vi "ztscopeM Download Record.vi"(0 "Instrument Handle In":i32, 1 "startTime":dbl format="%^#_6g", 5 "Source":i32(ring) items=["Input Channel 1", "Input Channel 2", "Input Channel 3", "Input Channel 4", "Calc Channel 1", "Calc Channel 2", "Calc Channel 3", "Calc Channel 4", "Ref Channel 1", "Ref Channel 2", "Ref Channel 3", "Ref Channel 4"], 7 "Points":i32=1000, 9 "Transfer Type":i32(ring)=2 items=["s8", "s16", "s32", "f32", "f64"], 11 "error in":errorcluster, 12 "stopTime":dbl format="%^#_6g") -> (3 "F64 Wave":dbl[](array[numeric]), 4 "Instrument Handle Out":i32, 6 "S8 Wave":i8[](array[numeric]), 8 "S16 Wave":i16[](array[numeric]), 10 "S32 Wave":i32[](array[numeric]), 14 "F32 Wave":sgl[](array[numeric]), 15 "error out":errorcluster)   [LabVIEW 2013]
doc: "Read the waveform in the source channel. The returned data format depends on the Transfer Type. Use \"Read Waveform Preamble\" to get the appropriate time and magnitude bases."
uses:
  ztscopeM.dll
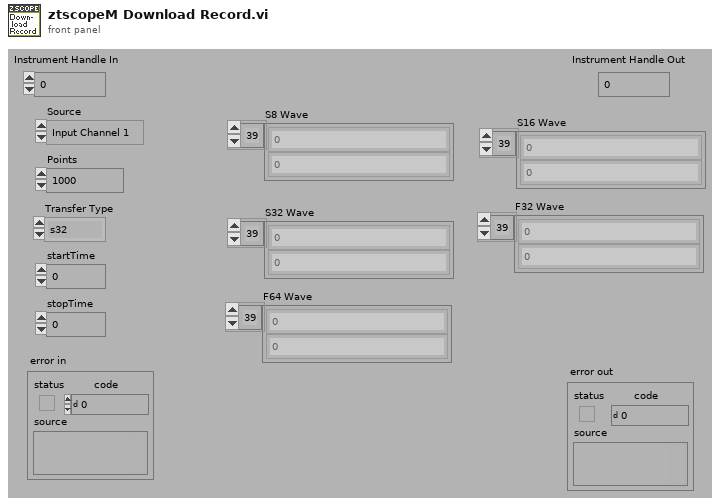
[diagram p1: front panel]
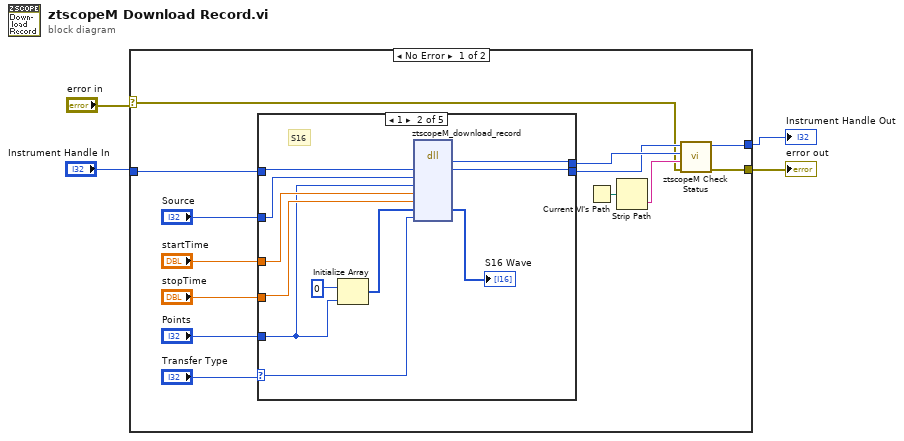
[diagram p0: block diagram]
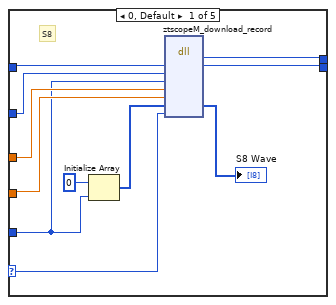
[diagram p2: hidden frame]
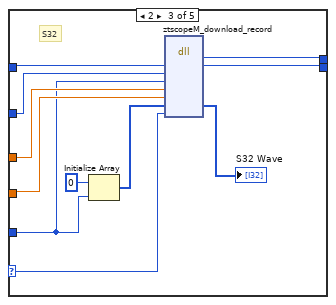
[diagram p3: hidden frame]
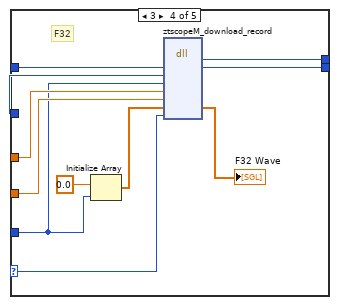
[diagram p4: hidden frame]
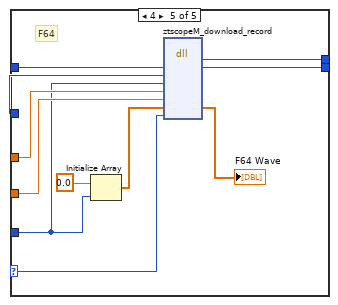
[diagram p5: hidden frame]
diagram:
  n1 = case shown="No Error" "error in" {
    selector: "error in" -> [w10 w74]
    tunnel: [w12 w74] -> w1
    tunnel: "Instrument Handle In" -> [w11 w73]
    tunnel: [w13 w73] -> w3
    frame No Error {
      n2 = case shown="1" "Transfer Type" {
        selector: "Transfer Type" -> [w19 w30 w41 w52 w63]
        tunnel: [w21 w32 w43 w60 w71] -> w15
        tunnel: [w20 w31 w42 w59 w70] -> w14
        tunnel: w11 -> [w22 w33 w44 w58 w69]
        tunnel: "Points" -> [w18 w29 w40 w51 w62]
        tunnel: "Source" -> [w23 w34 w45 w57 w68]
        tunnel: "startTime" -> [w24 w35 w46 w54 w65]
        tunnel: "stopTime" -> [w25 w36 w47 w53 w64]
        frame 0, Default {
          # "S8"
          n3 = Initialize Array(i8 0, w18) -> (w27:i8[])
          n4 = dll-call lib="C:/Program Files/National Instruments/instr.lib/ztscopem/ztscopeM.dll" fn="ztscopeM_download_record"("instrumentHandle"=w22, "source"=w23, "points"=w18, "startTime"=w24, "stopTime"=w25, "Waveform"=w27, "transferType"=w19) -> (w21:i32, "instrumentHandle"=w20:i32, "Waveform"=→"S8 Wave":i8[])  [unwired: 8 in, 2 out]
        }
        frame 1 {
          # "S16"
          n5 = Initialize Array(i16 0, w29) -> (w38:i16[])
          n6 = dll-call lib="C:/Program Files/National Instruments/instr.lib/ztscopem/ztscopeM.dll" fn="ztscopeM_download_record"("instrumentHandle"=w33, "source"=w34, "points"=w29, "startTime"=w35, "stopTime"=w36, "Waveform"=w38, "transferType"=w30) -> (w32:i32, "instrumentHandle"=w31:i32, "Waveform"=→"S16 Wave":i16[])  [unwired: 8 in, 2 out]
        }
        frame 2 {
          # "S32"
          n7 = Initialize Array(0, w40) -> (w49:i32[])
          n8 = dll-call lib="C:/Program Files/National Instruments/instr.lib/ztscopem/ztscopeM.dll" fn="ztscopeM_download_record"("instrumentHandle"=w44, "source"=w45, "points"=w40, "startTime"=w46, "stopTime"=w47, "Waveform"=w49, "transferType"=w41) -> (w43:i32, "instrumentHandle"=w42:i32, "Waveform"=→"S32 Wave":i32[])  [unwired: 8 in, 2 out]
        }
        frame 3 {
          # "F32"
          n9 = Initialize Array(sgl 0.0, w51) -> (w56:sgl[])
          n10 = dll-call lib="C:/Program Files/National Instruments/instr.lib/ztscopem/ztscopeM.dll" fn="ztscopeM_download_record"("instrumentHandle"=w58, "source"=w57, "points"=w51, "startTime"=w54, "stopTime"=w53, "Waveform"=w56, "transferType"=w52) -> (w60:i32, "instrumentHandle"=w59:i32, "Waveform"=→"F32 Wave":sgl[])  [unwired: 8 in, 2 out]
        }
        frame 4 {
          # "F64"
          n11 = Initialize Array(0.0, w62) -> (w67:dbl[])
          n12 = dll-call lib="C:/Program Files/National Instruments/instr.lib/ztscopem/ztscopeM.dll" fn="ztscopeM_download_record"("instrumentHandle"=w69, "source"=w68, "points"=w62, "startTime"=w65, "stopTime"=w64, "Waveform"=w67, "transferType"=w63) -> (w71:i32, "instrumentHandle"=w70:i32, "Waveform"=→"F64 Wave":dbl[])  [unwired: 8 in, 2 out]
        }
      }
      n13 = Current VI's Path() -> (path=w17:path)
      n14 = Strip Path(path=w17) -> (name=w16:string)  [unwired: 1 out]
      n15 = call "ztscopeM Check Status.vi"("error in"=w10, "name of VI"=w16, "status"=w15, "instrument handle in"=w14) -> ("error out"=w12:errorcluster, "instrument handle out"=w13:i32)  [unwired: 2 in]
    }
    frame Error {
    }
  }
  "Instrument Handle Out" <- w3
  "error out" <- w1
